vi "FINS CMD Get Info.vi"(10 "CMD in":T1) -> (0 "Bytes":string, 2 "CMD out":T1)   [LabVIEW 2019, in "FINS TCP.lvlib"]
uses:
  FINS TCP.lvlib
  FINS CMD.ctl
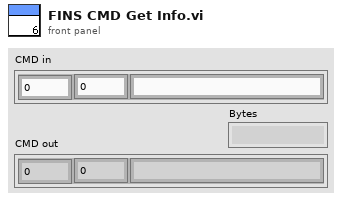
[diagram p1: front panel]
types:
  T1 = typedef "FINS TCP.lvlib/FINS CMD.ctl" = cluster{"MR":u8, "SR":u8, "name":string}
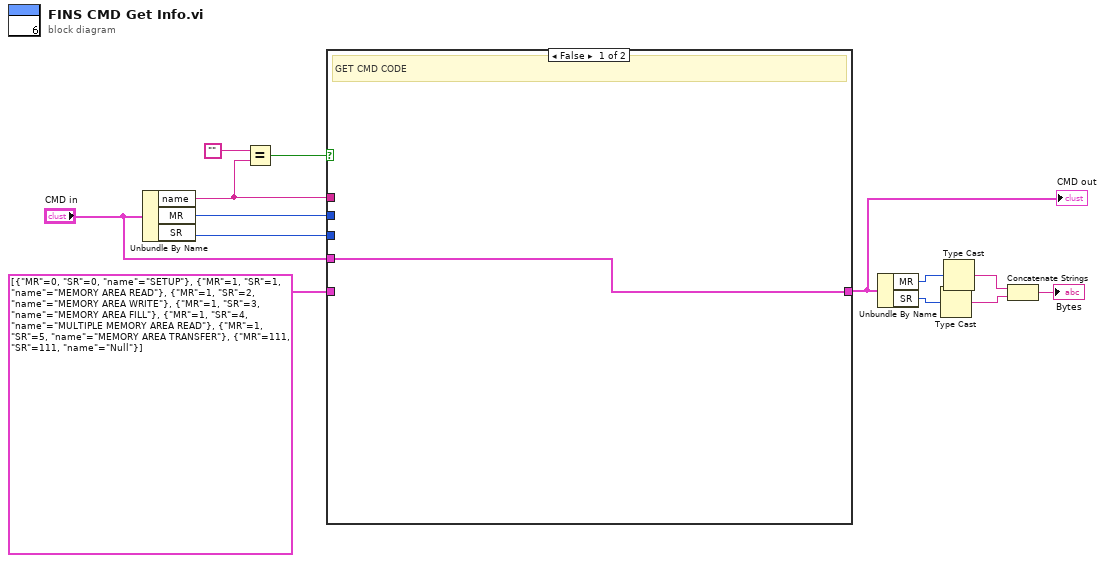
[diagram p0: block diagram]
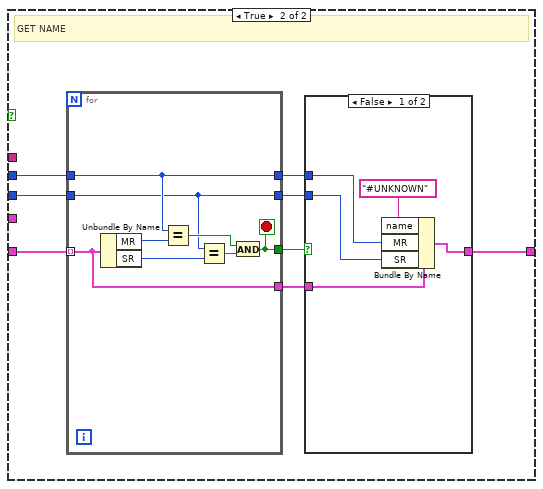
[diagram p2: hidden frame]
diagram:
  n1 = Unbundle By Name("CMD in") -> ("name"=w10:string, "MR"=w12:u8, "SR"=w11:u8)
  n2 = Equal?(x="", y=w10) -> (x = y?=w8:bool)
  n3 = case shown="False" w8 {
    tunnel: T1[] [{"MR"=0, "SR"=0, "name"="SETUP"}, {"MR"=1, "SR"=1, "name"="MEMORY AREA READ"}, {"MR"=1, "SR"=2, "name"="MEMORY AREA WRITE"}, {"MR"=1, "SR"=3, "name"="MEMORY AREA FILL"}, {"MR"=1, "SR"=4, "name"="MULTIPLE MEMORY AREA READ"}, {"MR"=1, "SR"=5, "name"="MEMORY AREA TRANSFER"}, {"MR"=111, "SR"=111, "name"="Null"}] -> [_ w22]
    tunnel: w10 -> [_ _]
    tunnel: w12 -> [_ w21]
    tunnel: w11 -> [_ w20]
    tunnel: [w14 w15] -> w2
    tunnel: "CMD in" -> [w14 _]
    frame False {
      # "GET CMD CODE"
    }
    frame True {
      # "GET NAME"
      n4 = for {
        tunnel: w22 -> [w32] mode=indexing
        tunnel: w21 -> [w30]
        tunnel: w20 -> [w29]
        tunnel: [w32] -> w19
        tunnel: [w31] -> w18
        tunnel: [w30] -> w17
        tunnel: [w29] -> w16
        stop <- w31 stop-if-true
        n5 = Unbundle By Name(w32) -> ("MR"=w36:u8, "SR"=w35:u8)
        n6 = Equal?(x=w30, y=w36) -> (x = y?=w34:bool)
        n7 = Equal?(x=w29, y=w35) -> (x = y?=w33:bool)
        n8 = And(x=w34, y=w33) -> (x .and. y?=w31:bool)
      }
      n9 = case shown="False" w18 {
        tunnel: w19 -> [w27 w28]
        tunnel: w17 -> [w26 _]
        tunnel: w16 -> [w25 _]
        tunnel: [w24 w28] -> w15
        frame False {
          n10 = Bundle By Name(cluster=w27, "name"="#UNKNOWN", "MR"=w26, "SR"=w25) -> (w24:T1)
        }
        frame True {
        }
      }
    }
  }
  "CMD out" <- w2
  n11 = Unbundle By Name(w2) -> ("MR"=w3:u8, "SR"=w4:u8)
  n12 = Type Cast(x=w4) -> (*(type *) &x=w6:string)  [unwired: 1 in]
  n13 = Type Cast(x=w3) -> (*(type *) &x=w7:string)  [unwired: 1 in]
  n14 = Concatenate Strings(w7, w6) -> (→"Bytes":string)
